vi "liblinxdevice Path.vi"(0 "Path":path, 1 "Operation":T1=enum."Get") -> (6 "Lib Path":path)   [LabVIEW 2014, in "LMH-LINX.lvlib" / "Local IO.lvlib"]
uses:
  <vilib>/MakerHub/LINX/Private/Local IO/Local IO.lvlib
  <vilib>/MakerHub/LINX/Private/Type Defs/FGV Operation.ctl
  <vilib>/MakerHub/LINX/LMH-LINX.lvlib
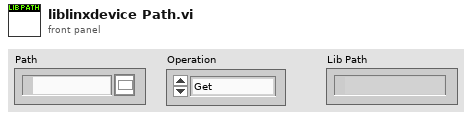
[diagram p1: front panel]
types:
  T1 = typedef "LMH-LINX.lvlib/FGV Operation.ctl" = enum16{"Initialize", "Get", "Set"}
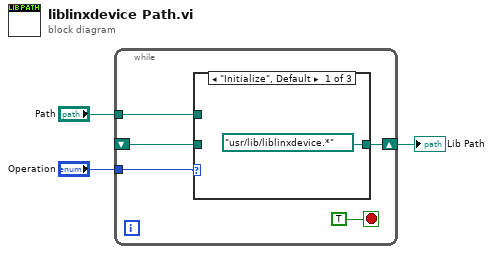
[diagram p0: block diagram]
diagram:
  n1 = while {
    tunnel: "Operation" -> [w7]
    shift-right: [w6] -> w1
    shift-left: _ -> [w5]
    tunnel: "Path" -> [w4]
    stop <- TRUE stop-if-true
    n2 = case shown="\"Initialize\", Default" w7 {
      tunnel: [path "/usr/lib/liblinxdevice.*" w10 w11] -> w6
      tunnel: w5 -> [_ w10 _]
      tunnel: w4 -> [_ _ w11]
      frame "Initialize", Default {
      }
      frame "Get" {
      }
      frame "Set" {
      }
    }
  }
  "Lib Path" <- w1
